vi "Write function name.vi"(8 "error in (no error)":errorcluster, 10 "function name":string, 11 "User.Python in":refnum<class "User.Python.lvclass">) -> (0 "error out":errorcluster, 3 "User.Python out":refnum<class "User.Python.lvclass">)   [LabVIEW 2019, in "User.Python.lvclass"]
doc: "Write function name."
uses:
  User.Python.lvclass
  User.Python.lvclass/User.Python.ctl
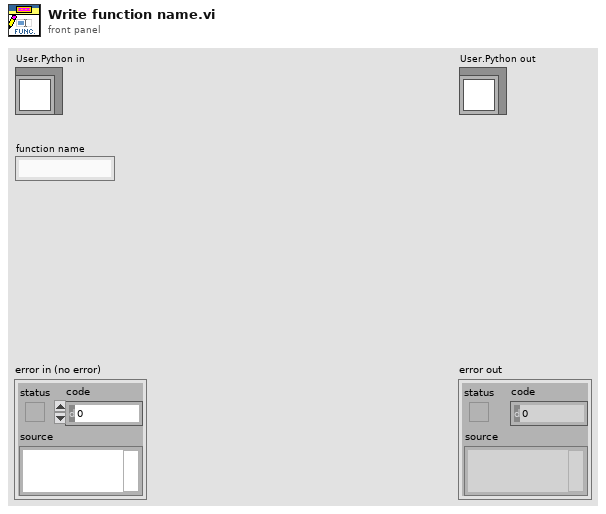
[diagram p1: front panel]
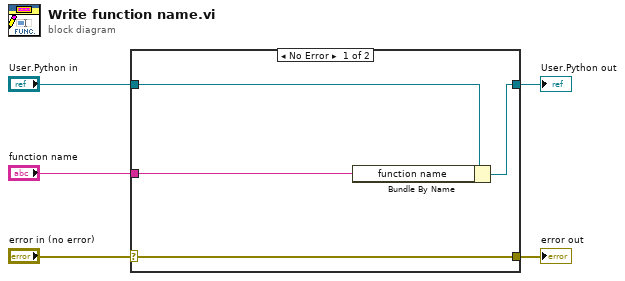
[diagram p0: block diagram]
diagram:
  n1 = case shown="No Error" "error in (no error)" {
    selector: "error in (no error)" -> [w9 w10]
    tunnel: [w9 w10] -> w4
    tunnel: [w7 w11] -> w2
    tunnel: "User.Python in" -> [w8 w11]
    tunnel: "function name" -> [w6 _]
    frame No Error {
      n2 = Bundle By Name(cluster=w8, "function name"=w6) -> (w7:refnum<class "User.Python.lvclass">)
    }
    frame Error {
    }
  }
  "error out" <- w4
  "User.Python out" <- w2
